vi "Quadrature.vi"(6 "Reset Counter":bool, 7 "Quad A":bool, 8 "ticks in":i32, 9 "Last Quad B":bool, 10 "Last Quad A":bool, 11 "Quad B":bool) -> (3 "ticks out":i32)   [LabVIEW 2015]
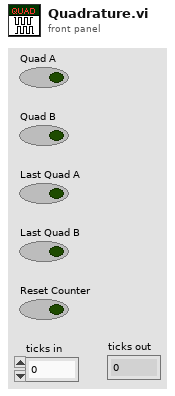
[diagram p1: front panel]
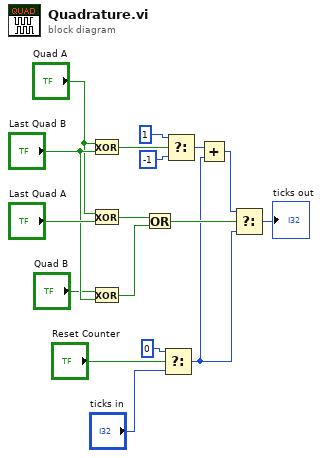
[diagram p0: block diagram]
diagram:
  n1 = Exclusive Or(1:"Last Quad B", 2:"Quad A") -> (0:w11:bool)
  n2 = Exclusive Or(1:"Last Quad A", 2:"Quad A") -> (0:w6:bool)
  n3 = Exclusive Or(1:"Last Quad B", 2:"Quad B") -> (0:w5:bool)
  n4 = Or(x=w6, y=w5) -> (x .or. y?=w7:bool)
  n5 = Select(t=0, s="Reset Counter", f="ticks in") -> (s? t:f=w2:i32)
  n6 = Select(t=1 ("x"), s=w11, f=-1 ("x")) -> (s? t:f=w9:i32)
  n7 = Add(x=w9, y=w2) -> (x+y=w1:i32)
  n8 = Select(t=w1, s=w7, f=w2) -> (s? t:f=→"ticks out":i32)
